vi "Write TDM Event Data.vi"() -> ()   [LabVIEW 2023]
doc: "Simulates a continuous data acquisition in a loop. The data values are appended to a single data channel. During the simulated measurement, random events will cause the VI to calculate a histogram on the most recent data package and to store it to a new data channel. Two additional data channels are created to store time stamps of the event occurrences and text descriptions of the events."
uses:
  <vilib>/Platform/storage/lvStorage.llb/_openFunction.ctl
  <vilib>/Platform/storage/Storage.llb/usiSequenceRepresentation.ctl
  <vilib>/Platform/storage/Storage.llb/usiOverwriteOptions.ctl
  <vilib>/Platform/storage/lvStorage.llb/_openStorageWithRootAutoDetect.vi
  <vilib>/Platform/storage/lvStorage.llb/xStorage/xStorageSupp/ErrorOut.vi
  Instance           2 24Saved   Write Event Data .vi
  <vilib>/Platform/storage/lvStorage.llb/_createOrGetExplicitChildObject.vi
  <vilib>/Platform/storage/lvStorage.llb/_prepDDT.vi
  <vilib>/Platform/storage/lvStorage.llb/_getChannelNameFromDDT.vi
  <vilib>/Platform/storage/lvStorage.llb/_createOrGetByNameExplicitChildObject.vi
  <vilib>/Platform/storage/lvStorage.llb/_saveDDT.vi
  <vilib>/Platform/storage/Storage.llb/__savePropString.vi
  <vilib>/Platform/storage/lvStorage.llb/__saveInt32Channel.vi
  <vilib>/Platform/storage/lvStorage.llb/__saveStringChannel.vi
  <vilib>/Platform/storage/Storage.llb/Get Object Info.vi
  <vilib>/Platform/storage/Storage.llb/__closeStorageFromObject.vi
  <vilib>/Platform/storage/lvStorage.llb/xStorage/Open Data Storage/Open Data Storage.xnode
  <vilib>/Platform/storage/lvStorage.llb/xStorage/Write Data/Write Data.xnode
  <vilib>/Platform/storage/lvStorage.llb/xStorage/Close Data Storage/Close Data Storage.xnode
panel:
  out "Current Data":dynamicdata(graph)
  # "Overview: Demonstrates the use of the DataPlugin Express VIs to write event data to a TDM file.\nRequirements: Windows\nInstructions:\n1. Run this VI.\n2. Open Read TDM Event Data.vi and follow the instructions on its front panel."
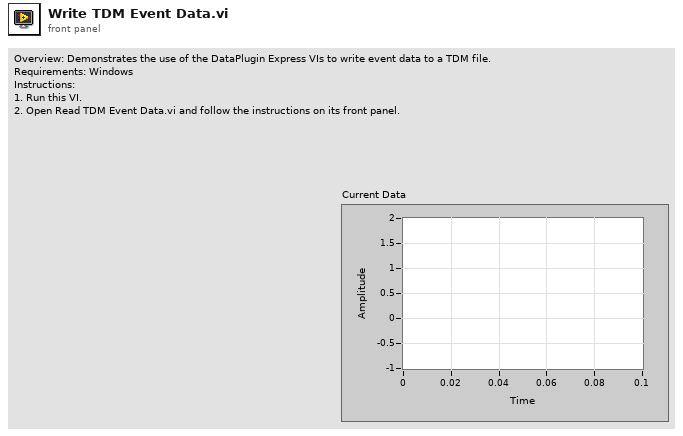
[diagram p1: front panel]
types:
  T1 = enum16{"UPDATE", "READ", "QUERY", "CREATE CHILD", "CREATE", "CONNECT", "DISCONNECT"}
  T2 = typedef "usiOverwriteOptions.ctl" = enum16{"Append values", "Replace values at index", "Replace all values", "Append if timeline aligns"}
  T3 = typedef "usiSequenceRepresentation.ctl" = enum16{"explicit", "implicit"}
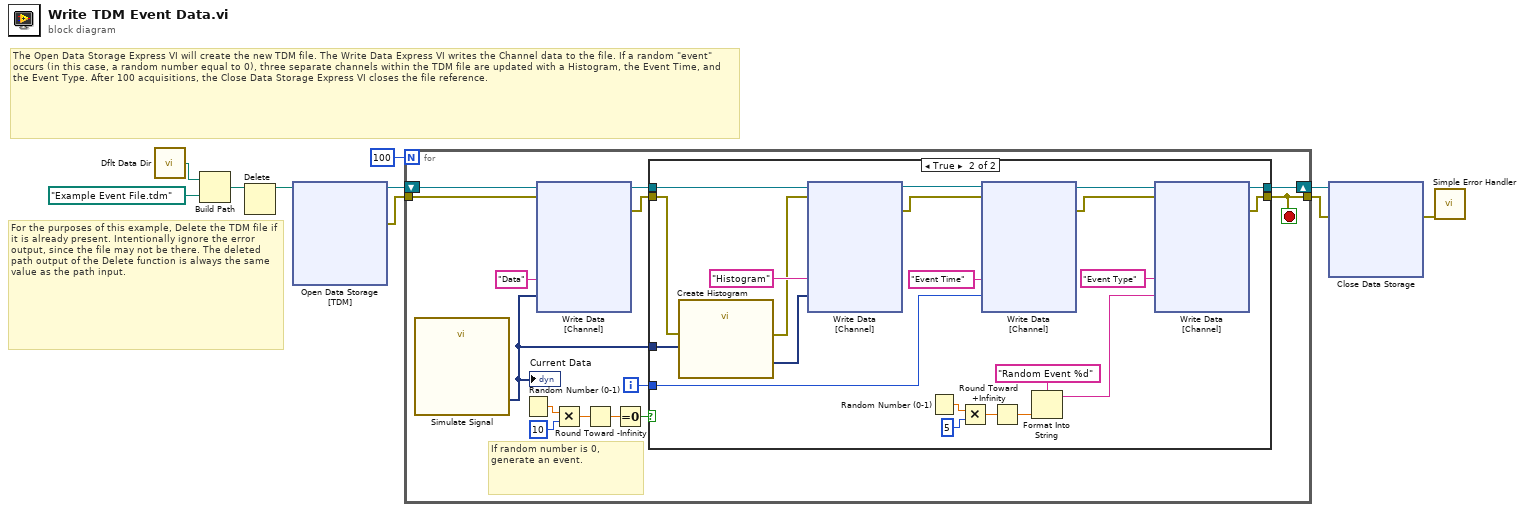
[diagram p0: block diagram]
diagram:
  # "The Open Data Storage Express VI will create the new TDM file. The Write Data Express VI writes the Channel data to the file. If a random \"event\" occurs (in this case, a random number equal to 0), three separate channels within the TDM file are updated with a Histogram, the Event Time, and the Event Type. After 100 acquisitions, the Close Data Storage Express VI closes the file reference."
  # "For the purposes of this example, Delete the TDM file if it is already present. Intentionally ignore the error output, since the file may not be there. The deleted path output of the Delete function is always the same value as the path input."
  n1 = call <vilib>:"Dflt Data Dir.vi"() -> ("App:Default Data Directory"=w2:path)
  n2 = Build Path(base path=w2, name or relative path=path "Example Event File.tdm" ("default name")) -> (appended path=w4:path)
  n3 = Delete(path (use dialog)=w4) -> (deleted path=w1:path)  [unwired: 4 in, 2 out]
  n4 = xnode "Open Data Storage\n[TDM]"("file path"=w1) -> ("storage refnum (file)"=w7:refnum<k20>, "error out"=w6:errorcluster)  [unwired: 2 in, 3 out]
  n5 = for {
    N: 100 -> [_]
    tunnel: w6 -> [w22]
    tunnel: [w18] -> w8
    shift-right: [w19] -> w9
    shift-left: w7 -> [w23]
    i -> [w24]
    stop <- w18 stop-if-true
    # "If random number is 0, generate an event."
    n6 = call "Simulate Signal"() -> ("Sine with Noise"=w12:dynamicdata)  [unwired: 8 in, 7 out]
    "Current Data" <- w12
    n7 = Random Number (0-1)() -> (number: 0 to 1=w16:dbl)
    n8 = xnode "Write Data\n[Channel]"("Name"="Data" ("registertxt3"), "Signal"=w12, "storage refnum (file)"=w23, "error in"=w22) -> ("storage refnum (file) out"=w21:refnum<k20>, "error out"=w20:errorcluster)  [unwired: 3 out]
    n9 = Multiply(x=w16, y=10) -> (x*y=w14:dbl)
    n10 = Round Toward -Infinity(1:w14) -> (0:w17:dbl)
    n11 = Equal To 0?(x=w17) -> (x = 0?=w13:bool)
    n12 = case shown="True" w13 {
      tunnel: w12 -> [_ w70]
      tunnel: w24 -> [_ w62]
      tunnel: w21 -> [w58 w79]
      tunnel: w20 -> [w57 w60]
      tunnel: [w58 w72] -> w19
      tunnel: [w57 w71] -> w18
      frame False {
      }
      frame True {
        n13 = call "Create Histogram"("error in (no error)"=w60, "Signal"=w70) -> ("error out"=w59:errorcluster, "Histogram"=w69:dynamicdata)  [unwired: 3 in, 5 out]
        n14 = xnode "Write Data\n[Channel]"("Name"="Histogram" ("registertxt3"), "Signal"=w69, "storage refnum (file)"=w79, "error in"=w59) -> ("storage refnum (file) out"=w78:refnum<k20>, "error out"=w77:errorcluster)  [unwired: 2 in, 1 out]
        n15 = Random Number (0-1)() -> (number: 0 to 1=w68:dbl)
        n16 = Multiply(x=w68, y=5) -> (x*y=w66:dbl)
        n17 = xnode "Write Data\n[Channel]"("Name"="Event Time" ("name"), "Signal"=w62, "storage refnum (file)"=w78, "error in"=w77) -> ("storage refnum (file) out"=w74:refnum<k20>, "error out"=w73:errorcluster)  [unwired: 3 out]
        n18 = Round Toward +Infinity(x=w66) -> (ceil(x): smallest int >= x=w65:dbl)
        n19 = Format Into String(format string="Random Event %d", w65) -> (resulting string=w63:string)  [unwired: 2 in, 1 out]
        n20 = xnode "Write Data\n[Channel]"("Name"="Event Type" ("name"), "Signal"=w63, "storage refnum (file)"=w74, "error in"=w73) -> ("storage refnum (file) out"=w72:refnum<k20>, "error out"=w71:errorcluster)  [unwired: 3 out]
      }
    }
  }
  n21 = xnode "Close Data Storage\n"("storage refnum (file)"=w9, "error in (no error)"=w8) -> ("error out"=w5:errorcluster)  [unwired: 1 out]
  n22 = call <vilib>:"Simple Error Handler.vi"("error in (no error)"=w5) -> ()  [unwired: 1 in, 8 out]
